vi "COMI US Change Scan Freq.vi"(10 "dwScanFreq":u32, 11 "hDevice":u32) -> (2 "function return":i32, 3 "hDevice out":u32)   [LabVIEW 2017, in "Comidll.lvlib"]
doc: "long (COMI_US_ChangeScanFreq) (HANDLE hDevice, unsigned int dwScanFreq);"
uses:
  <userlib>/Comidll/Comidll.lvlib
  <userlib>/Comidll/Comidll.dll
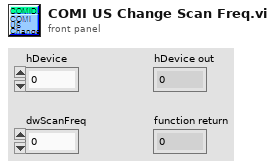
[diagram p1: front panel]
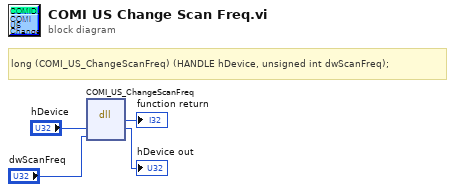
[diagram p0: block diagram]
diagram:
  # "long\t(COMI_US_ChangeScanFreq) (HANDLE hDevice, unsigned int dwScanFreq);"
  n1 = dll-call lib="C:/Program Files/National Instruments/LabVIEW 2017/user.lib/Comidll/Comidll.*" fn="COMI_US_ChangeScanFreq"("hDevice"="hDevice", "dwScanFreq"="dwScanFreq") -> (→"function return":i32, "hDevice"=→"hDevice out":u32)  [unwired: 4 in, 2 out]
